vi "OnDrop.vi"(0 "XRef":T7, 1 "State In":T1 {"BlockNodeState"."Draw Style" items=["FunctionBlock", "ExpressVI", "Variable", "Elemental I/O", "32x32 Icon", "FunctionBlockCompact"]; "BlockNodeState"."Terminal Data"."Terminal Flags" format="%.0b"}) -> (14 "Reply":T5, 16 "State Out":T1 {"BlockNodeState"."Draw Style" items=["FunctionBlock", "ExpressVI", "Variable", "Elemental I/O", "32x32 Icon", "FunctionBlockCompact"]; "BlockNodeState"."Terminal Data"."Terminal Flags" format="%.0b"})   [LabVIEW 2017, in "NI_Robotics_Create Steering Frame.xnode"]
uses:
  <vilib>/robotics/Steering/Create Steering Frame/NI_Robotics_Create Steering Frame.xnode
  <vilib>/XNodeSupport/XNodeXNodeRef.ctl
  <vilib>/robotics/Steering/Create Steering Frame/State.ctl
  <vilib>/BlockNodeSupport/BlockNodeState.ctl
  <vilib>/BlockNodeSupport/TerminalData.ctl
  <vilib>/picture/picture.llb/imagedata.ctl
  <vilib>/XNodeSupport/XNodeStringArray.ctl
  <vilib>/XNodeSupport/XNodeString.ctl
  <vilib>/XNodeSupport/NI_XNodeSupport.lvlib
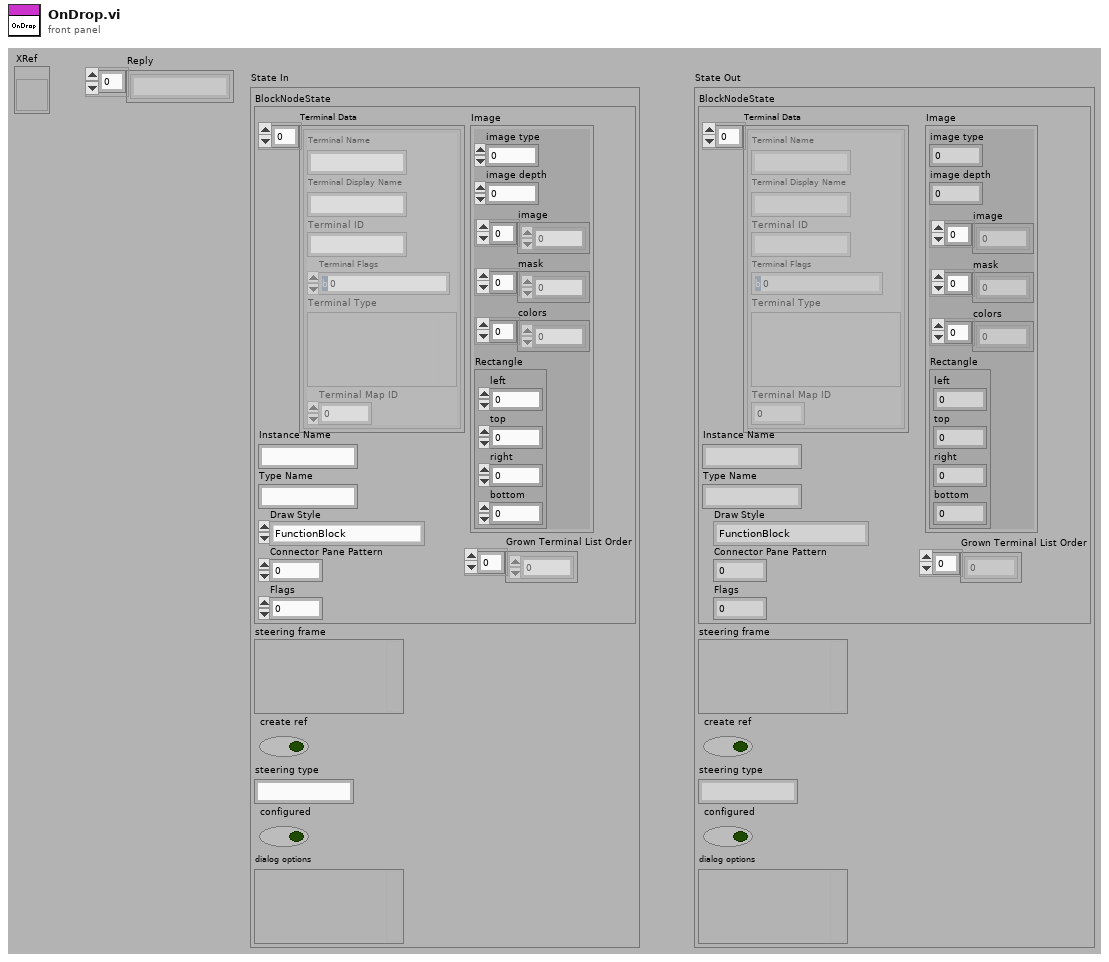
[diagram p1: front panel]
types:
  T1 = typedef "NI_Robotics_Create Steering Frame.xnode/State.ctl" = cluster{"BlockNodeState":T2, "steering frame":variant, "create ref":bool, "steering type":string, "configured":bool, "dialog options":variant}
  T2 = typedef "BlockNodeState.ctl" = cluster{"Terminal Data":T3[], "Instance Name":string, "Type Name":string, "Draw Style":i32, "Connector Pane Pattern":i32, "Flags":i32, "Grown Terminal List Order":i32[], "Image":T4}
  T3 = typedef "TerminalData.ctl" = cluster{"Terminal Name":string, "Terminal Display Name":string, "Terminal ID":string, "Terminal Flags":i32, "Terminal Type":variant, "Terminal Map ID":i32}
  T4 = typedef "imagedata.ctl" = cluster{"image type":i32, "image depth":i32, "image":u8[], "mask":u8[], "colors":u32[], "Rectangle":cluster{"left":i16, "top":i16, "right":i16, "bottom":i16}}
  T5 = typedef "NI_XNodeSupport.lvlib/XNodeStringArray.ctl" = T6[]
  T6 = typedef "NI_XNodeSupport.lvlib/XNodeString.ctl" = string
  T7 = typedef "NI_XNodeSupport.lvlib/XNodeXNodeRef.ctl" = refnum<vi>
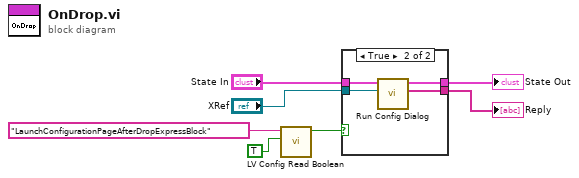
[diagram p0: block diagram]
diagram:
  n1 = call <resource>:"LV Config Read Boolean.vi"("default value"=TRUE, "key"="LaunchConfigurationPageAfterDropExpressBlock") -> ("value"=w1:bool)  [unwired: 3 in, 2 out]
  n2 = case shown="True" w1 {
    tunnel: "State In" -> [w8 w12]
    tunnel: [_ w11] -> w6
    tunnel: "XRef" -> [_ w10]
    tunnel: [w8 w9] -> w4
    frame False {
    }
    frame True {
      n3 = call <vilib>:"Run Config Dialog.vi"("XRef"=w10, "State In"=w12) -> ("Reply"=w11:T5, "State Out"=w9:T1)  [unwired: 7 in, 1 out]
    }
  }
  "Reply" <- w6
  "State Out" <- w4
